vi "Ask Theta.vi"(8 "error in (no error)":errorcluster, 11 "Module in":refnum<class "Module.lvclass">) -> (0 "error out":errorcluster, 2 "Theta Error Out":dbl, 3 "Module out":refnum<class "Module.lvclass">)   [LabVIEW 2018, in "Module.lvclass"]
uses:
  Module.lvclass
  Module.lvclass/Module.ctl
panel:
  out "Tray Position":dbl
  out "Tray Region":dbl
  out "Tray Number":dbl
  in  "Submit":bool
  in  "Theta Error (OGP)":dbl
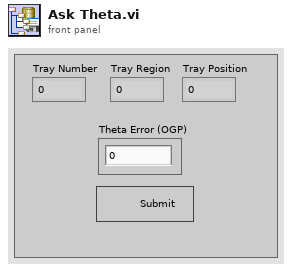
[diagram p1: front panel]
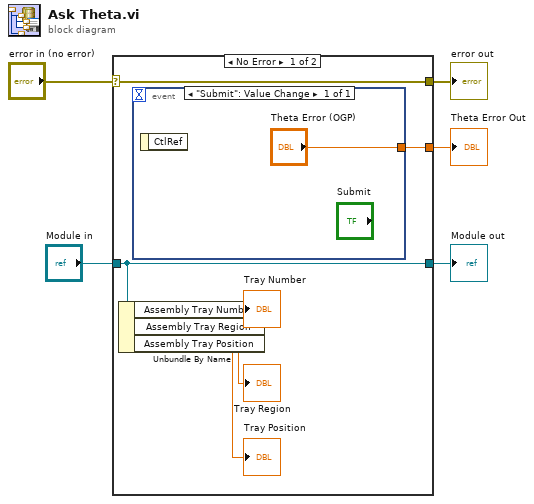
[diagram p0: block diagram]
diagram:
  n1 = case shown="No Error" "error in (no error)" {
    selector: "error in (no error)" -> [w11 w14]
    tunnel: [w11 w14] -> w4
    tunnel: [w10 w13] -> w2
    tunnel: "Module in" -> [w10 w13]
    tunnel: [w6 _] -> w1
    frame No Error {
      n2 = Unbundle By Name(w10) -> ("Assembly Tray Number"=→"Tray Number":dbl, "Assembly Tray Region"=→"Tray Region":dbl, "Assembly Tray Position"=→"Tray Position":dbl)
      n3 = event shown="[0] \"Submit\": Value Change" {
        selector: _ -> [_]
        dyn-events: _ -> [_]
        timeout: _ -> [_]
        tunnel: ["Theta Error (OGP)"] -> w6
        event "Submit": Value Change {
          n4 = event-data() -> ()  [unwired: 1 in, 1 out]
        }
      }
    }
    frame Error {
    }
  }
  "error out" <- w4
  "Module out" <- w2
  "Theta Error Out" <- w1
